vi "SetScales.vi"(9 "Sleep":u32, 11 "XYGraph in":refnum<vi>) -> (1 "Sleep":u32)   [LabVIEW 2025]
uses:
  Globals.vi
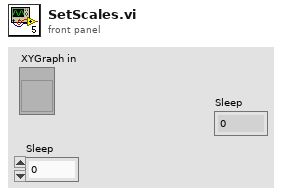
[diagram p1: front panel]
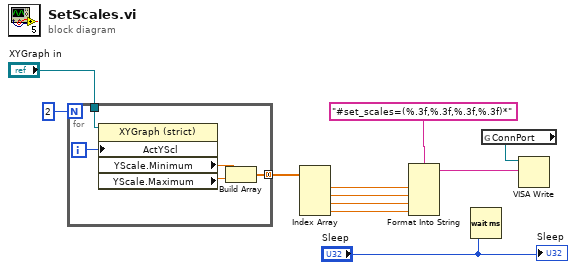
[diagram p0: block diagram]
diagram:
  n1 = for {
    N: 2 -> [_]
    tunnel: [w16] -> w5 mode=concatenating
    tunnel: "XYGraph in" -> [w15]
    i -> [w12]
    n2 = property class="XYGraph (strict)"(reference=w15, "ActYScl"=w12) -> ("YScale.Minimum"=w14:dbl, "YScale.Maximum"=w13:dbl)  [unwired: 1 in, 2 out]
    n3 = Build Array(w14, w13) -> (w16:dbl[])
  }
  n4 = Index Array(array=w5) -> (element #1=w6:dbl, element #2=w2:dbl, element #3=w7:dbl, element #4=w8:dbl)  [unwired: 4 in]
  n5 = Format Into String(format string="#set_scales=(%.3f,%.3f,%.3f,%.3f)*", w6, w2, w7, w8) -> (resulting string=w9:string)  [unwired: 2 in, 1 out]
  n6 = Wait (ms)(milliseconds to wait="Sleep") -> ()  [unwired: 1 out]
  n7 = global read "Globals.vi" "ConnPort"() -> (w10:refnum<visa-resource-name>)
  n8 = VISA Write(VISA resource name=w10, write buffer=w9) -> ()  [unwired: 1 in, 3 out]
  "Sleep" <- "Sleep"
